vi "Read Default Object Cluster.vi"(8 "error in (no error)":errorcluster, 11 "ObjectSettings in":refnum<class "ObjectSettings.lvclass">) -> (0 "error out":errorcluster, 2 "Default Object":T1, 3 "ObjectSettings out":refnum<class "ObjectSettings.lvclass">)   [LabVIEW 2019, in "ObjectSettings.lvclass"]
uses:
  ObjectSettings.lvclass
  Typedefs/DefaultCluster.ctl
  ObjectSettings.lvclass/ObjectSettings.ctl
  <vilib>/JDP Science/JSONtext/JSONtext.lvlib
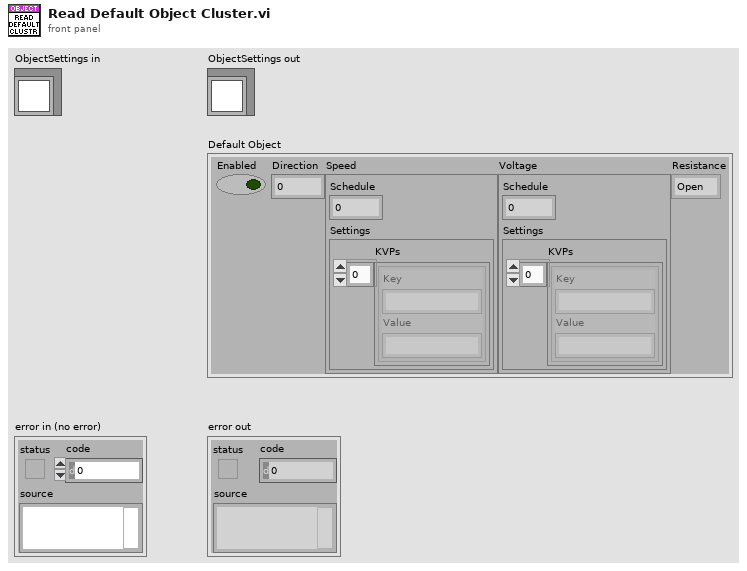
[diagram p1: front panel]
types:
  T1 = typedef "ObjectSettings.lvclass/DefaultCluster.ctl" = cluster{"Enabled":bool, "Direction":u16, "Speed":cluster{"Schedule":u16, "Settings":cluster{"KVPs":cluster{"Key":string, "Value":string}[]}}, "Voltage":cluster{"Schedule":u16, "Settings":cluster{"KVPs":cluster{"Key":string, "Value":string}[]}}, "Resistance":enum16{"Open", "Discharge Tip", "0 ohm", "100 kohm", "10 Mohm", "1 Gohm"}}
  T2 = enum16{"Open", "Discharge Tip", "0 ohm", "100 kohm", "10 Mohm", "1 Gohm"}
  T3 = cluster{cluster{"substring":string, "<JSON>":string}[]}
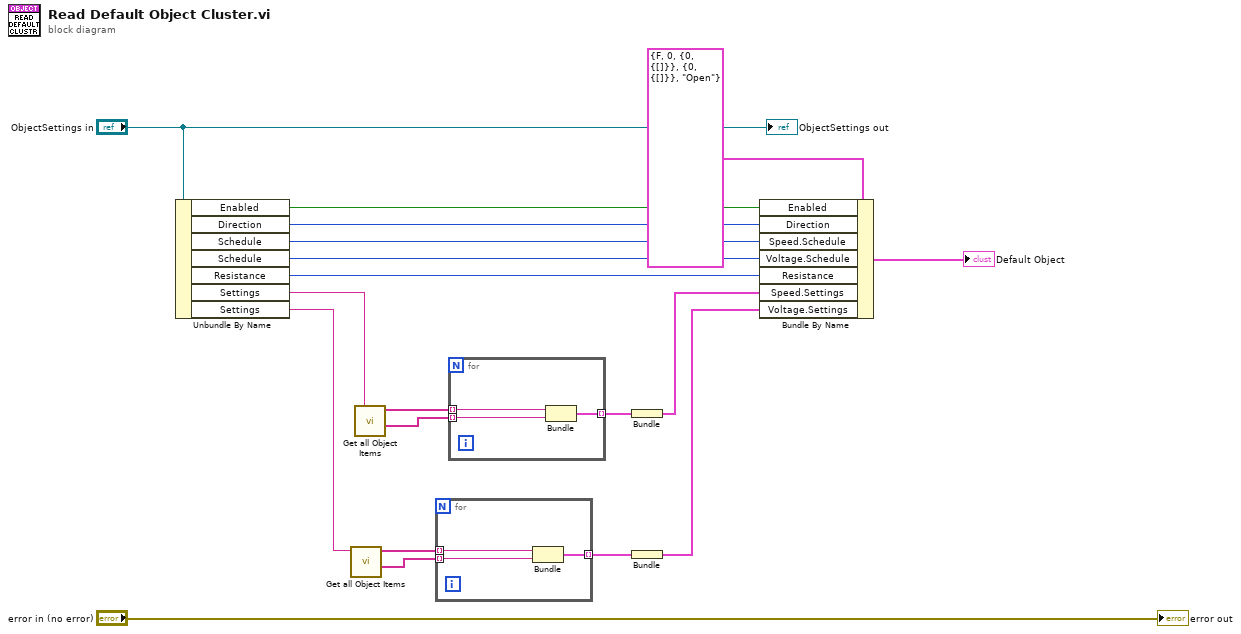
[diagram p0: block diagram]
diagram:
  n1 = Unbundle By Name("ObjectSettings in") -> ("Enabled"=w18:bool, "Direction"=w17:u16, "Schedule"=w12:u16, "Schedule"=w11:u16, "Resistance"=w15:T2, "Settings"=w3:string, "Settings"=w6:string)
  n2 = call <vilib>:"Get all Object Items.vi"("JSON"=w6) -> ("<JSON>"=w4:string[], "Item Names"=w5:string[])  [unwired: 7 in, 2 out]
  n3 = call <vilib>:"Get all Object Items.vi"("JSON"=w3) -> ("<JSON>"=w1:string[], "Item Names"=w2:string[])  [unwired: 7 in, 2 out]
  n4 = for {
    tunnel: w5 -> [w22] mode=indexing
    tunnel: w4 -> [w20] mode=indexing
    tunnel: [w21] -> w9 mode=indexing
    n5 = Bundle("substring"=w22, "<JSON>"=w20) -> (w21:cluster{"substring":string, "<JSON>":string})  [unwired: 1 in]
  }
  n6 = for {
    tunnel: w2 -> [w25] mode=indexing
    tunnel: w1 -> [w23] mode=indexing
    tunnel: [w24] -> w10 mode=indexing
    n7 = Bundle("substring"=w25, "<JSON>"=w23) -> (w24:cluster{"substring":string, "<JSON>":string})  [unwired: 1 in]
  }
  n8 = Bundle(w10) -> (w7:T3)  [unwired: 1 in]
  n9 = Bundle(w9) -> (w8:T3)  [unwired: 1 in]
  n10 = Bundle By Name(cluster=T1 {"Enabled"=FALSE, "Direction"=0, "Speed"={"Schedule"=0, "Settings"={"KVPs"=[]}}, "Voltage"={"Schedule"=0, "Settings"={"KVPs"=[]}}, "Resistance"=enum."Open"}, "Enabled"=w18, "Direction"=w17, "Speed.Schedule"=w12, "Voltage.Schedule"=w11, "Resistance"=w15, "Speed.Settings"=w7, "Voltage.Settings"=w8) -> (→"Default Object":T1)
  "error out" <- "error in (no error)"
  "ObjectSettings out" <- "ObjectSettings in"
